vi "ES Main.vi"(10 "Data Type DVRs":T1, 11 "Config Folder":path) -> ()   [LabVIEW 2018]
uses:
  <vilib>/ORNL/CSEISMIC DDS/CSEISMIC DDS Base/Data Types/Controls/DeviceID.ctl
  Controls/DDS State.ctl
  Controls/Data Type DVRs.ctl
  Controls/Generation Mode Loop Selector.ctl
  <vilib>/ORNL/CSEISMIC DDS/CSEISMIC DDS Base/Data Types/DER_setGenerationMode.ctl
  <vilib>/ORNL/CSEISMIC DDS/CSEISMIC DDS Base/Data Types/Controls/Generation Mode.ctl
  Controls/GenerationMode.ctl
  <vilib>/ORNL/CSEISMIC DDS/CSEISMIC DDS Base/Data Types/IED_Status.ctl
  <vilib>/ORNL/CSEISMIC DDS/CSEISMIC DDS Base/Data Types/Controls/Timestamp.ctl
  <vilib>/ORNL/CSEISMIC DDS/CSEISMIC DDS Base/Data Types/DER_Control.ctl
  <vilib>/ORNL/CSEISMIC DDS/CSEISMIC DDS Base/Data Types/DER_SetPointP.ctl
  <vilib>/ORNL/CSEISMIC DDS/CSEISMIC DDS Base/Data Types/DER_SetPointQ.ctl
  <vilib>/ORNL/CSEISMIC DDS/CSEISMIC DDS Base/Data Types/DER_SetPointV.ctl
  <vilib>/ORNL/CSEISMIC DDS/CSEISMIC DDS Base/Data Types/DER_VF.ctl
  <vilib>/ORNL/CSEISMIC DDS/CSEISMIC DDS Base/Data Types/DER_SetPointF.ctl
  <vilib>/ORNL/CSEISMIC DDS/CSEISMIC DDS Base/Data Types/DER_Measurement.ctl
  <vilib>/ORNL/CSEISMIC DDS/CSEISMIC DDS Base/Data Types/DER_Status.ctl
  <vilib>/ORNL/CSEISMIC DDS/CSEISMIC DDS Base/Data Types/Controls/DroopCurve.ctl
  <vilib>/ORNL/CSEISMIC DDS/CSEISMIC DDS Base/Data Types/ES_Measurement.ctl
  c0909f76-96e0-496f-a6f7-ac9c3abfbcaa.vi
  7c59bdfa-a6d0-42ea-a36a-6a540bb37f3e.vi
  e95f3c18-e29d-40e4-94d7-6429cff7ece6.vi
  5e6c5b3f-77aa-4a8f-ba55-705d5b229056.vi
  7d30dc78-1fe7-43d0-be68-14ef1da03709.vi
  d3906dff-0d56-43f1-806b-b312a818046b.vi
  60710d3d-d05d-4e06-abc4-5833922697d4.vi
  d723711c-90b5-43fd-9837-430fe65d8763.vi
  2b29db2b-b629-43ef-99c9-7f779e92d8e6.vi
  fb202ae5-af77-46d5-8a34-636558cc811c.vi
  de1367b4-29ab-415d-92d0-7fa0fc6667ea.vi
  a8c78b73-a0ab-4721-a181-3ce0dcbdf431.vi
  9b782105-9e9e-450c-bef0-451d1281a5e4.vi
  04e9c7aa-85a8-4273-86f5-9355a9113040.vi
  f60448c4-0b4d-4df0-bc80-4b02817c393f.vi
  ae97810f-c92e-4387-8c39-39f975af07db.vi
  Global Variables/Stop (Global).vi
  Global Variables/Measurements (Global).vi
  Global Variables/DDS States (Global).vi
  Global Variables/Manual Control (Global).vi
  <vilib>/ORNL/CSEISMIC DDS/CSEISMIC DDS Base/CSEISMIC DDS.lvclass
panel:
  out "P_ref":sgl
  out "Q_ref":sgl
  out "P_meas":sgl
  out "Vf Control":bool
  out "Q_meas":sgl
  out "f_islanded":fxp<+,20,6>
  out "Vq_ref":sgl
  out "5038 Count":u32
  out "Is VF Device?":bool
  in  "Ramp Rate (W)":sgl=5000.0
  out "MicrogridID":u8
  out "Error in DDS Loop":bool
  out "DDS Loop error out":errorcluster
  out "DDS State":T2=enum."Shutdown"
  out "DDS loop time":u32=103
  out "DDS Indicators":T3
  out "Error in Generation Mode Loop":bool
  out "error out GenMode Loop":errorcluster
  out "DDS state m/c loop time":u32=100
  out "DeviceID":T4
  out "Enable INV A":bool
  out "SOC":dbl
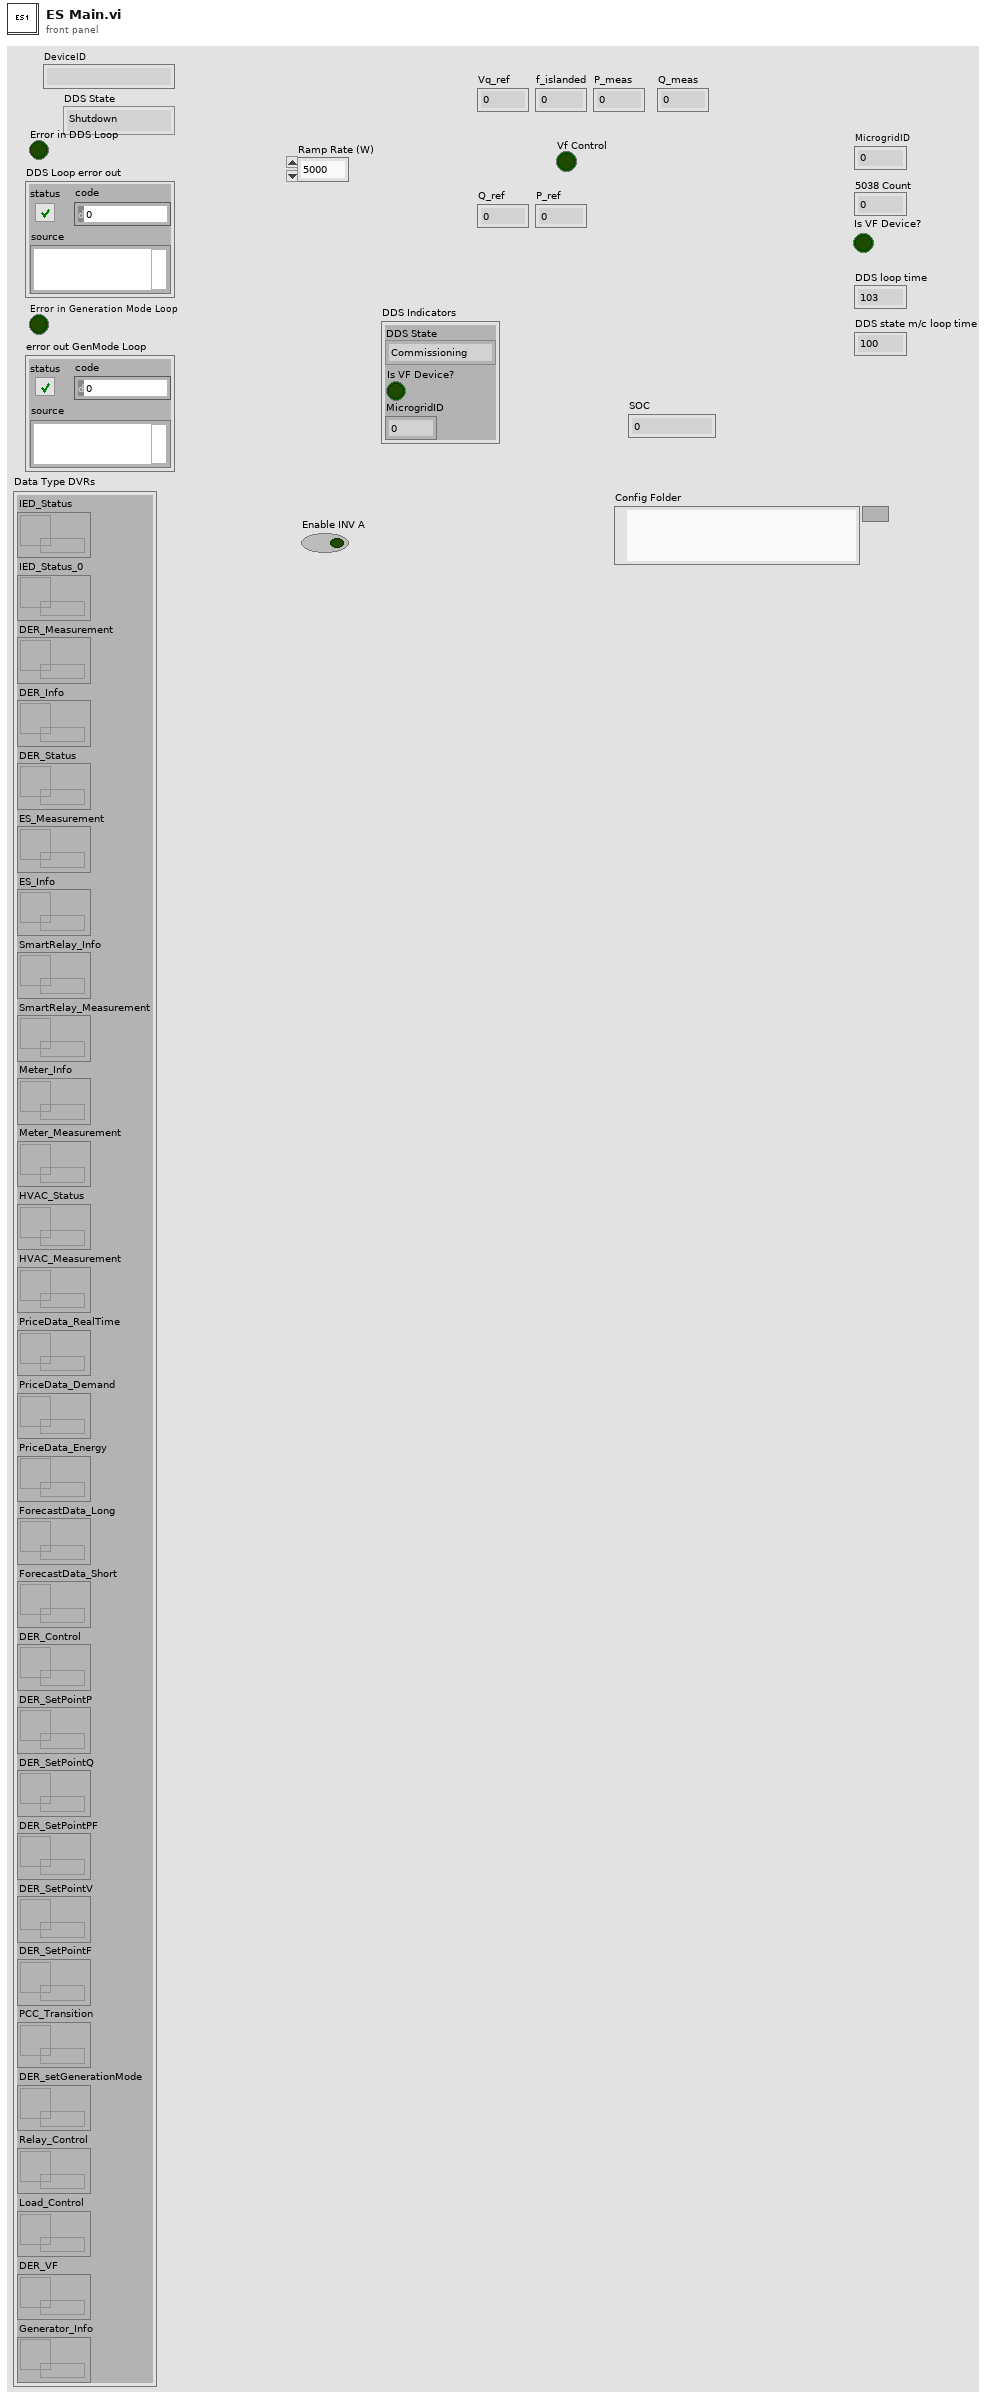
[diagram p1: front panel]
types:
  T1 = typedef "Data Type DVRs.ctl" = cluster{"IED_Status":refnum<data-value>, "IED_Status_0":refnum<data-value>, "DER_Measurement":refnum<data-value>, "DER_Info":refnum<data-value>, "DER_Status":refnum<data-value>, "ES_Measurement":refnum<data-value>, "ES_Info":refnum<data-value>, "SmartRelay_Info":refnum<data-value>, "SmartRelay_Measurement":refnum<data-value>, "Meter_Info":refnum<data-value>, "Meter_Measurement":refnum<data-value>, "HVAC_Status":refnum<data-value>, "HVAC_Measurement":refnum<data-value>, "PriceData_RealTime":refnum<data-value>, "PriceData_Demand":refnum<data-value>, "PriceData_Energy":refnum<data-value>, "ForecastData_Long":refnum<data-value>, "ForecastData_Short":refnum<data-value>, "DER_Control":refnum<data-value>, "DER_SetPointP":refnum<data-value>, "DER_SetPointQ":refnum<data-value>, "DER_SetPointPF":refnum<data-value>, "DER_SetPointV":refnum<data-value>, "DER_SetPointF":refnum<data-value>, "PCC_Transition":refnum<data-value>, "DER_setGenerationMode":refnum<data-value>, "Relay_Control":refnum<data-value>, "Load_Control":refnum<data-value>, "DER_VF":refnum<data-value>, "Generator_Info":refnum<data-value>}
  T2 = typedef "DDS State.ctl" = enum16{"Commissioning", "CheckID", "InitDDS", "ReadDDS", "WriteDDS", "CheckClose", "Close", "Shutdown"}
  T3 = cluster{"DDS State":T2, "Is VF Device?":bool, "MicrogridID":u8}
  T4 = typedef "CSEISMIC DDS.lvlib/CSEISMIC DDS.lvclass/DeviceID.ctl" = string
  T5 = typedef "Generation Mode Loop Selector.ctl" = enum16{"Commissioning", "Start", "Active", "VF Device", "Hold", "Close References", "Shutdown"}
  T6 = typedef "Scaling Coefficients Cluster.ctl" = cluster{"Measurements":T7, "Setpoints":T8}
  T7 = typedef "Scaling Coefficients Measurements.ctl" = cluster{"Current":dbl, "Voltage":dbl, "Real Power":dbl, "Reactive Power":dbl, "SOC":dbl}
  T8 = typedef "Scaling Coefficients Setpoints.ctl" = cluster{"Voltage":dbl, "Frequency":dbl, "Real Power":dbl, "Reactive Power":dbl}
  T9 = typedef "CSEISMIC DDS.lvlib/CSEISMIC DDS.lvclass/DER_Info.ctl" = cluster{"DeviceID":T4, "LineConfig":u8[], "NominalVoltage(V)":dbl, "PowerRating(kVA)":dbl, "VFControl":bool, "PControl":bool, "QControl":bool, "PFControl":bool, "PVControl":bool, "Droop":bool, "DroopConfigurable":bool, "Unbalanced":bool}
  T10 = typedef "CSEISMIC DDS.lvlib/CSEISMIC DDS.lvclass/ES_Info.ctl" = cluster{"DeviceID":T4, "EnergyRating (kWh)":dbl, "RampRate (kW/s)":dbl, "MaxPowerFactorLeading":dbl, "MaxPowerFactorLagging":dbl, "ChargingEfficiencyCurve":T11, "DischargingEfficiencyCurve":T11, "MinSOC (%)":dbl, "MaxSOC (%)":dbl}
  T11 = typedef "CSEISMIC DDS.lvlib/CSEISMIC DDS.lvclass/EfficiencyCurve.ctl" = cluster{"Power (kW)":dbl[], "Efficiency (%)":dbl[]}
  T12 = typedef "CSEISMIC DDS.lvlib/CSEISMIC DDS.lvclass/DER_setGenerationMode.ctl" = cluster{"DeviceID":T4, "Mode":T13}
  T13 = typedef "CSEISMIC DDS.lvlib/CSEISMIC DDS.lvclass/Generation Mode.ctl" = enum32{"Invalid", "PQ", "Droop", "PV", "PF", "VF"}
  T14 = typedef "GenerationMode.ctl" = enum32{"Invalid", "PQ", "Droop", "PV", "PF", "VF"}
  T15 = typedef "CSEISMIC DDS.lvlib/CSEISMIC DDS.lvclass/Timestamp.ctl" = cluster{"Seconds":u64, "Remainder":u64}
  T16 = typedef "CSEISMIC DDS.lvlib/CSEISMIC DDS.lvclass/IED_Status.ctl" = cluster{"DeviceID":T4, "Timestamp":T15, "MicrogridID":u8, "Active":bool, "Inactive":bool, "Error":i32, "Fault":bool, "ErrorString":string}
  T17 = typedef "CSEISMIC DDS.lvlib/CSEISMIC DDS.lvclass/DER_SetPointF.ctl" = cluster{"DeviceID":T4, "Frequency (Hz)":dbl}
  T18 = typedef "CSEISMIC DDS.lvlib/CSEISMIC DDS.lvclass/DER_VF.ctl" = cluster{"DeviceID":T4}
  T19 = typedef "CSEISMIC DDS.lvlib/CSEISMIC DDS.lvclass/DER_SetPointV.ctl" = cluster{"DeviceID":T4, "Voltage (V)":dbl}
  T20 = typedef "CSEISMIC DDS.lvlib/CSEISMIC DDS.lvclass/DER_SetPointQ.ctl" = cluster{"DeviceID":T4, "ReactivePower (kVAR)":dbl[]}
  T21 = typedef "CSEISMIC DDS.lvlib/CSEISMIC DDS.lvclass/DER_SetPointP.ctl" = cluster{"DeviceID":T4, "RealPower (kW)":dbl[]}
  T22 = typedef "CSEISMIC DDS.lvlib/CSEISMIC DDS.lvclass/DER_Control.ctl" = cluster{"DeviceID":T4, "Activate":bool, "Deactivate":bool}
  T23 = typedef "CSEISMIC DDS.lvlib/CSEISMIC DDS.lvclass/ES_Measurement.ctl" = cluster{"DeviceID":T4, "SOC (%)":dbl}
  T24 = typedef "CSEISMIC DDS.lvlib/CSEISMIC DDS.lvclass/DER_Status.ctl" = cluster{"DeviceID":T4, "VFControl":bool, "PControl":bool, "QControl":bool, "PFControl":bool, "PVControl":bool, "Droop":bool, "Unbalanced":bool, "MicrogridVF":bool, "RealDroop(kW)":T25, "ReactiveDroop(kVar)":T25}
  T25 = typedef "CSEISMIC DDS.lvlib/CSEISMIC DDS.lvclass/DroopCurve.ctl" = cluster{"XMin":dbl, "XMax":dbl, "YMin":dbl, "YMax":dbl}
  T26 = typedef "CSEISMIC DDS.lvlib/CSEISMIC DDS.lvclass/DER_Measurement.ctl" = cluster{"DeviceID":T4, "Voltage":dbl[], "Current":dbl[], "RealPower":dbl[], "ReactivePower":dbl[], "LineConfig":u8[], "Frequency":dbl}
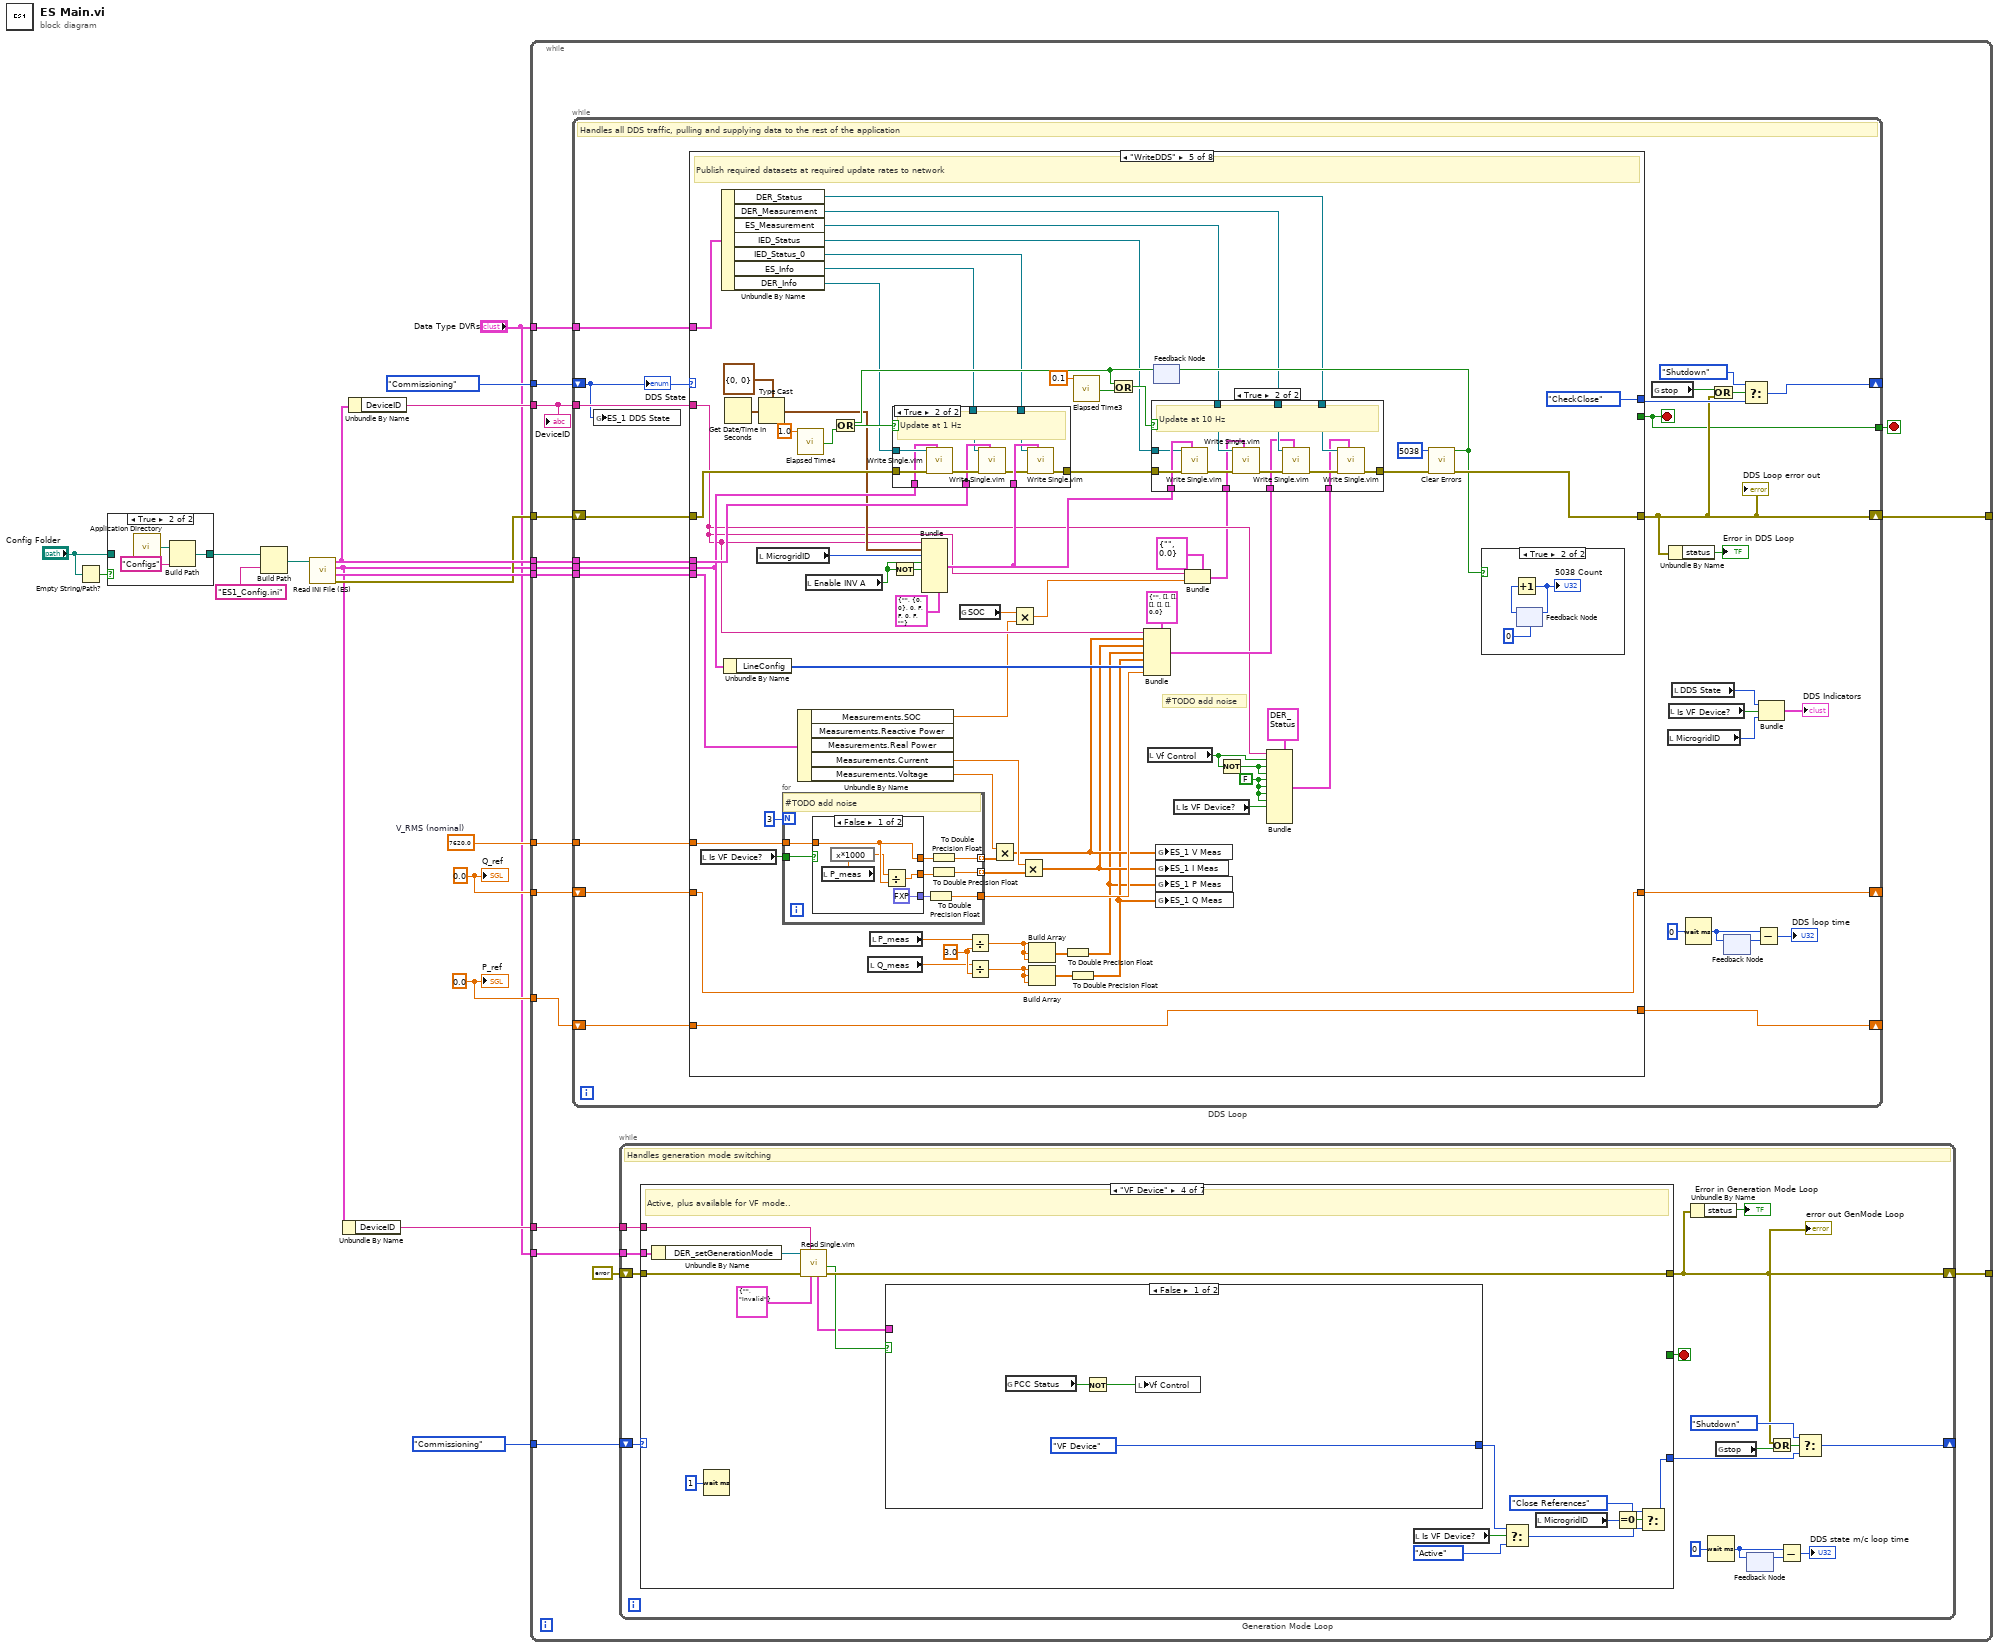
[diagram p0: block diagram]
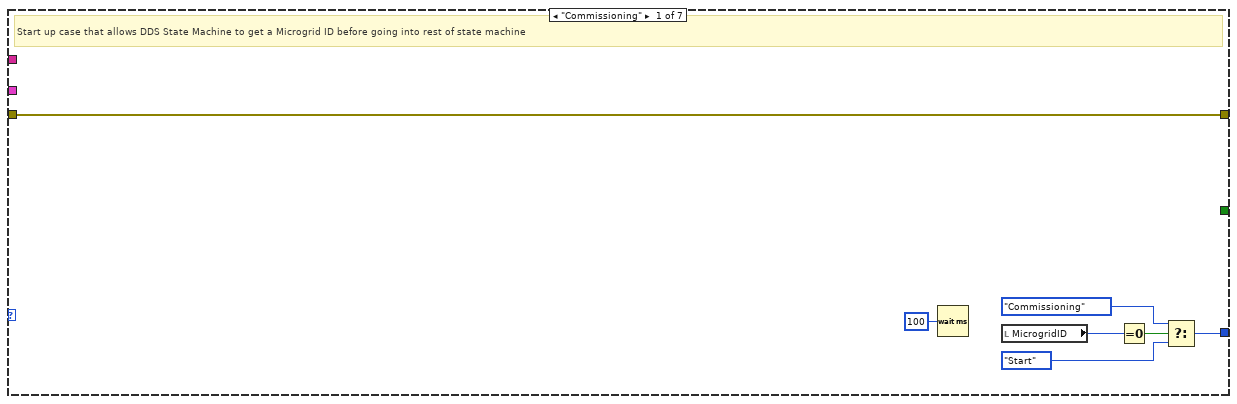
[diagram p2: hidden frame]
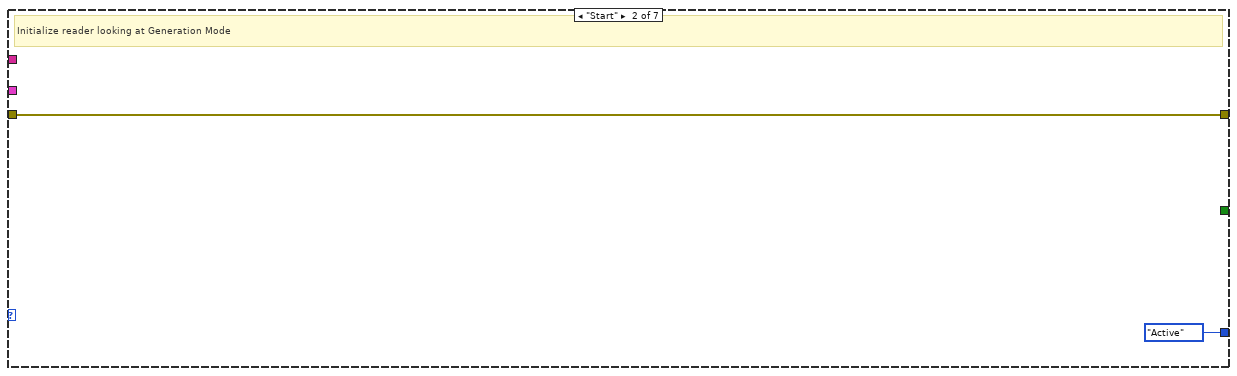
[diagram p3: hidden frame]
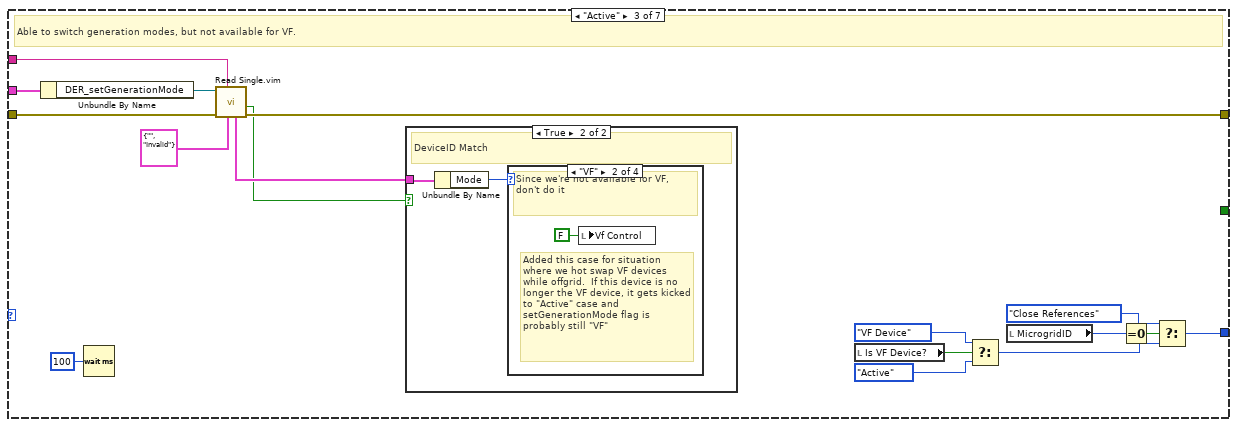
[diagram p4: hidden frame]
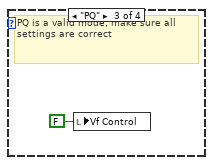
[diagram p7: hidden frame]
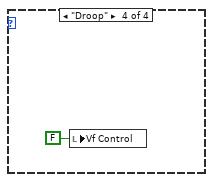
[diagram p8: hidden frame]
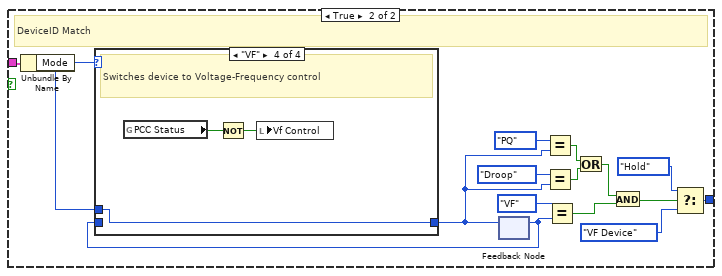
[diagram p9: hidden frame]
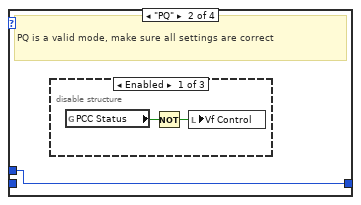
[diagram p11: hidden frame]
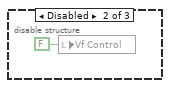
[diagram p12: hidden frame]
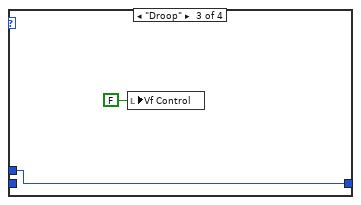
[diagram p14: hidden frame]
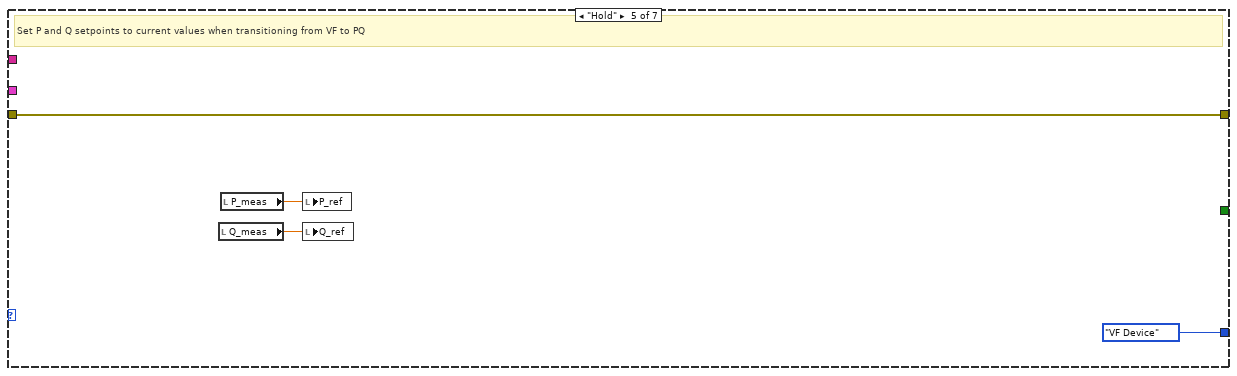
[diagram p15: hidden frame]
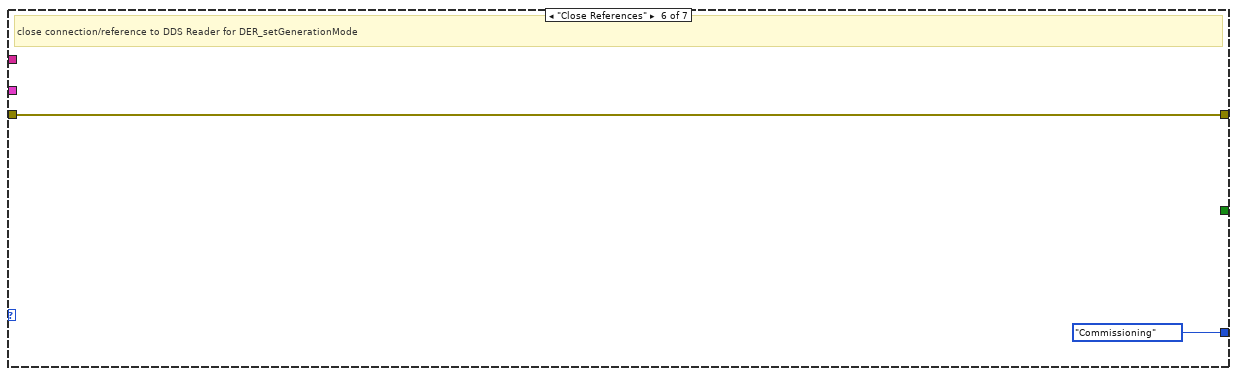
[diagram p16: hidden frame]
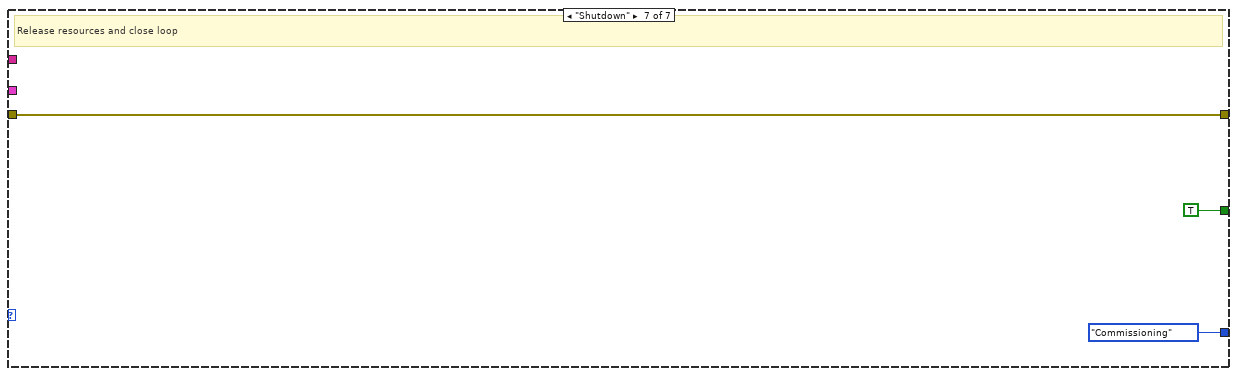
[diagram p17: hidden frame]
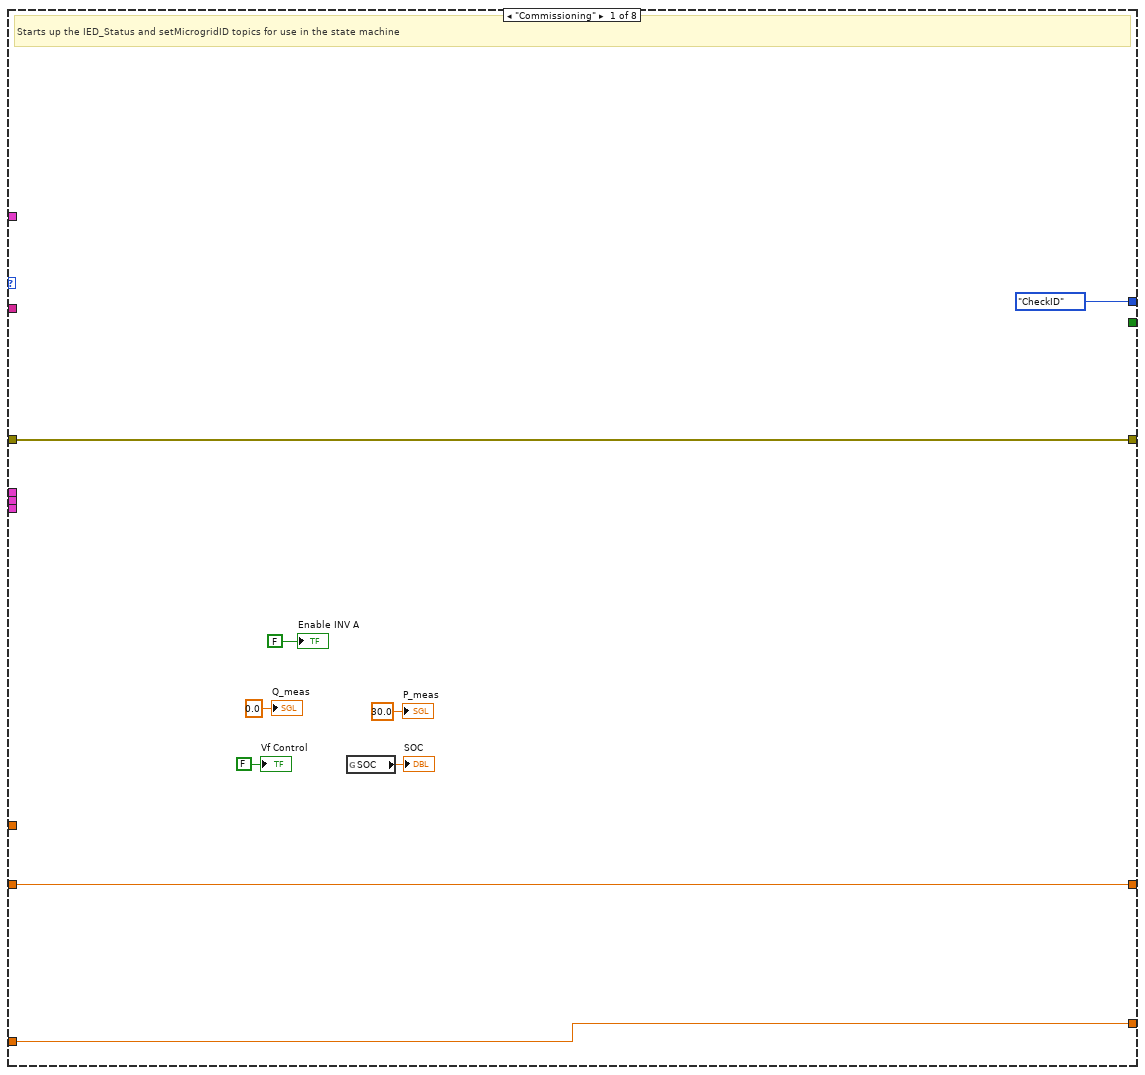
[diagram p18: hidden frame]
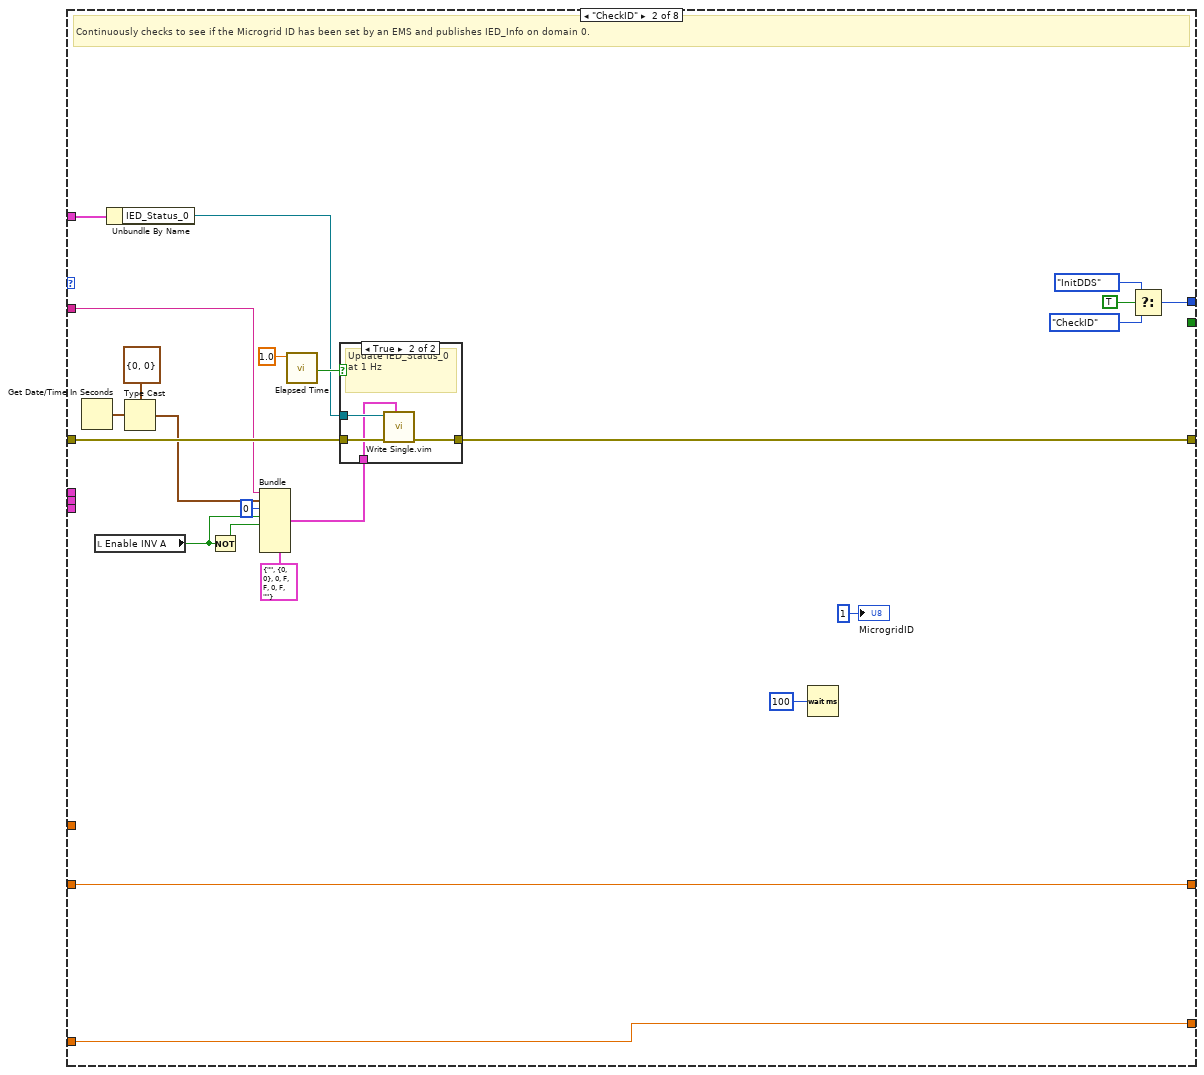
[diagram p19: hidden frame]
diagram:
  w5 = 7620.0  # V_RMS (nominal)
  w6 = sgl 0.0 ("Q_ref")
  w7 = sgl 0.0 ("P_ref")
  n1 = Empty String/Path?(string/path="Config Folder") -> (empty?=w4:bool)
  n2 = case shown="True" w4 {
    tunnel: [w18 w19] -> w2
    tunnel: "Config Folder" -> [w18 _]
    frame False {
    }
    frame True {
      n3 = call <vilib>:"Application Directory.vi"() -> ("Application Directory"=w21:path)
      n4 = Build Path(base path=w21, name or relative path="Configs") -> (appended path=w19:path)
    }
  }
  n5 = Build Path(base path=w2, name or relative path="ES1_Config.ini") -> (appended path=w16:path)
  n6 = call "Read INI File (ES).vi"("Path"=w16) -> ("error out"=w12:errorcluster, "Scaling Coefficients"=w13:T6, "DER_Info"=w10:T9, "ES_Info"=w14:T10)  [unwired: 7 in]
  n7 = Unbundle By Name(w10) -> ("DeviceID"=w11:T4)
  n8 = Unbundle By Name(w14) -> ("DeviceID"=w15:T4)
  n9 = while {
    tunnel: DDS_State."Commissioning" ("DDS State 2") -> [w38]
    tunnel: w10 -> [w37]
    tunnel: w12 -> [w36]
    tunnel: w13 -> [w35]
    tunnel: w15 -> [w34]
    tunnel: w14 -> [w33]
    tunnel: w11 -> [w31]
    tunnel: Generation_Mode_Loop_Selector."Commissioning" -> [w30]
    tunnel: [w29] -> _
    tunnel: [w28] -> _
    tunnel: w7 -> [w27]
    tunnel: w6 -> [w26]
    tunnel: w5 -> [w25]
    tunnel: "Data Type DVRs" -> [w24]
    tunnel: "Data Type DVRs" -> [w23]
    stop <- w32 stop-if-true
    n10 = while "DDS Loop" {
      shift-right: [w163] -> _
      shift-left: w38 -> [w140]
      tunnel: w34 -> [w167]
      shift-right: [w158] -> w28
      shift-left: w36 -> [w166]
      tunnel: w33 -> [w165]
      tunnel: w37 -> [w164]
      tunnel: w35 -> [w159]
      tunnel: [w156] -> w32
      shift-right: [w150] -> _
      shift-left: w27 -> [w149]
      shift-right: [w148] -> _
      shift-left: w26 -> [w147]
      tunnel: w25 -> [w142]
      tunnel: w24 -> [w151]
      stop <- w156 stop-if-true
      # "Handles all DDS traffic, pulling and supplying data to the rest of the application"
      n11 = global write "DDS States (Global).vi" "ES_1 DDS State"(w140) -> ()
      n12 = case shown="\"WriteDDS\"" w140 {
        tunnel: [DDS_State."CheckID" w194 DDS_State."ReadDDS" w254 DDS_State."CheckClose" w439 DDS_State."Commissioning" ("f") DDS_State."Commissioning" ("f")] -> w162
        tunnel: [w175 w185 w207 w221 w368 w438 w445 w452] -> w158
        tunnel: w167 -> [_ w184 _ w218 w353 _ _ _]
        tunnel: w166 -> [w175 w197 w207 w241 w387 w438 w445 w452]
        tunnel: w165 -> [_ _ _ _ w379 _ _ _]
        tunnel: w164 -> [_ _ _ _ w378 _ _ _]
        tunnel: [_ _ _ _ _ _ _ TRUE] -> w156
        tunnel: w159 -> [_ _ _ w210 w374 _ _ _]
        tunnel: w151 -> [_ w179 _ w242 w329 _ _ _]
        tunnel: [w174 w183 w206 w252 w346 w437 w443 w449] -> w150
        tunnel: w149 -> [w174 w183 w206 w251 w346 w437 w443 w449]
        tunnel: [w173 w182 w205 w249 w345 w436 w442 w448] -> w148
        tunnel: w147 -> [w173 w182 w205 w248 w345 w436 w442 w448]
        tunnel: w142 -> [_ _ _ _ w337 _ _ _]
        frame "Commissioning" {
          # "Starts up the IED_Status and setMicrogridID topics for use in the state machine"
          n13 = global read "Manual Control (Global).vi" "SOC"() -> (→"SOC":dbl)
          "Q_meas" <- sgl 0.0 ("Q_meas")
          "Vf Control" <- FALSE ("Vf Control")
          "P_meas" <- sgl 30.0 ("P_meas")
          "Enable INV A" <- FALSE ("Enable INV A")
        }
        frame "CheckID" {
          # "Continuously checks to see if the Microgrid ID has been set by an EMS and publishes IED_Info on domain 0."
          n14 = Get Date/Time In Seconds() -> (seconds since 1Jan1904=w190:timestamp)
          n15 = local read "Enable INV A"() -> (w181:bool)
          n16 = Unbundle By Name(w179) -> ("IED_Status_0"=w178:refnum<data-value>)
          n17 = Type Cast(type=T15 {"Seconds"=0, "Remainder"=0} ("Timestamp"), x=w190) -> (*(type *) &x=w188:T15)
          n18 = Not(x=w181) -> (.not. x?=w186:bool)
          n19 = Bundle(cluster=T16 {"DeviceID"="", "Timestamp"={"Seconds"=0, "Remainder"=0}, "MicrogridID"=0, "Active"=FALSE, "Inactive"=FALSE, "Error"=0, "Fault"=FALSE, "ErrorString"=""} ("output cluster"), "DeviceID"=w184, "Timestamp"=w188, "MicrogridID"=u8 0, "Active"=w181, "Inactive"=w186) -> (w198:T16)  [unwired: 3 in]
          n20 = call "Elapsed Time"("Time Target (s)"=1.0) -> ("Time has Elapsed"=w193:bool)  [unwired: 11 in, 7 out]
          n21 = case shown="True" w193 {
            tunnel: w198 -> [_ w201]
            tunnel: [w200 w202] -> w185
            tunnel: w197 -> [w200 w203]
            tunnel: w178 -> [_ w204]
            frame False {
            }
            frame True {
              # "Update IED_Status_0 at 1 Hz"
              n22 = call "Write Single.vim"("Data Element"=w201, "error in"=w203, "Data DVR"=w204) -> ("dup error out"=w202:errorcluster)  [unwired: 8 in]
            }
          }
          n23 = Wait (ms)(milliseconds to wait=u32 100) -> ()  [unwired: 1 out]
          n24 = Select(t=DDS_State."InitDDS", s=TRUE, f=DDS_State."CheckID") -> (s? t:f=w194:T2)
          "MicrogridID" <- u8 1 ("MicrogridID")
        }
        frame "InitDDS" {
          # "This initializes all readers and writers for DDS."
        }
        frame "ReadDDS" {
          # "Read device datasets from network and pass valid values to FPGA layer"
          n25 = Unbundle By Name(w242) -> ("DER_VF"=w217:refnum<data-value>, "DER_SetPointV"=w215:refnum<data-value>, "DER_SetPointF"=w226:refnum<data-value>, "DER_SetPointQ"=w230:refnum<data-value>, "DER_SetPointP"=w234:refnum<data-value>, "DER_Control"=w240:refnum<data-value>)
          n26 = call "Read Single.vim"("Data Type"=T22 {"DeviceID"="", "Activate"=FALSE, "Deactivate"=FALSE} ("DER_Control"), "DeviceID"=w218, "error in"=w241, "Data DVR"=w240) -> ("dup error out"=w236:errorcluster, "Valid"=w239:bool, "Data Element"=w238:T22)  [unwired: 5 in]
          n27 = call "Read Single.vim"("Data Type"=T21 {"DeviceID"="", "RealPower (kW)"=[]} ("DER_SetPointP"), "DeviceID"=w218, "error in"=w236, "Data DVR"=w234) -> ("dup error out"=w231:errorcluster, "Valid"=w233:bool, "Data Element"=w232:T21)  [unwired: 5 in]
          n28 = call "Read Single.vim"("Data Type"=T20 {"DeviceID"="", "ReactivePower (kVAR)"=[]} ("DER_SetPointQ"), "DeviceID"=w218, "error in"=w231, "Data DVR"=w230) -> ("dup error out"=w225:errorcluster, "Valid"=w228:bool, "Data Element"=w227:T20)  [unwired: 5 in]
          n29 = case shown="True" w233 {
            tunnel: w232 -> [_ w315]
            tunnel: w210 -> [_ w314]
            tunnel: [w295 w309] -> w252
            tunnel: w251 -> [w295 _]
            frame False {
              # "Non-matching DeviceID"
            }
            frame True {
              # "DeviceID matches this device"
              n30 = Unbundle By Name(w314) -> ("Setpoints.Real Power"=w312:dbl)
              n31 = Unbundle By Name(w315) -> ("RealPower (kW)"=w313:dbl[])
              n32 = global read "Measurements (Global).vi" "Load P Meas"() -> (w299:dbl[])
              n33 = global read "Measurements (Global).vi" "ES_2 P Meas"() -> (w303:dbl[])
              n34 = global read "Measurements (Global).vi" "Gen P Meas"() -> (w302:dbl[])
              n35 = global read "Measurements (Global).vi" "PV P Meas"() -> (w301:dbl[])
              n36 = Compound Arithmetic op=ADD(w303, w302, w301) -> (w300:dbl[])
              n37 = Add Array Elements(numeric array=w313) -> (sum=w311:dbl)
              n38 = Subtract(x=w300, y=w299) -> (x-y=w298:dbl[])
              n39 = Multiply(x=w312, y=w311) -> (x*y=w310:dbl)
              n40 = Add Array Elements(numeric array=w298) -> (sum=w296:dbl)
              n41 = local read "Enable INV A"() -> (w304:bool)
              n42 = local read "Vf Control"() -> (w305:bool)
              n43 = To Single Precision Float(number=w310) -> (single precision float=w307:sgl)
              n44 = To Single Precision Float(number=w296) -> (single precision float=w297:sgl)
              n45 = Select(t=w297, s=w305, f=w307) -> (s? t:f=w306:sgl)
              n46 = Select(t=w306, s=w304, f=sgl 0.0) -> (s? t:f=w309:sgl)
            }
          }
          n47 = case shown="True" w228 {
            tunnel: w227 -> [_ w294]
            tunnel: w210 -> [_ w293]
            tunnel: [w275 w285] -> w249
            tunnel: w248 -> [w275 _]
            frame False {
              # "Non-matching DeviceID"
            }
            frame True {
              # "DeviceID matches this device"
              n48 = Unbundle By Name(w293) -> ("Setpoints.Reactive Power"=w290:dbl)
              n49 = Unbundle By Name(w294) -> ("ReactivePower (kVAR)"=w292:dbl[])
              n50 = global read "Measurements (Global).vi" "Load Q Meas"() -> (w281:dbl[])
              n51 = global read "Measurements (Global).vi" "ES_2 Q Meas"() -> (w277:dbl[])
              n52 = global read "Measurements (Global).vi" "Gen Q Meas"() -> (w278:dbl[])
              n53 = global read "Measurements (Global).vi" "PV Q Meas"() -> (w279:dbl[])
              n54 = Compound Arithmetic op=ADD(w277, w278, w279) -> (w280:dbl[])
              n55 = Add Array Elements(numeric array=w292) -> (sum=w291:dbl)
              n56 = Subtract(x=w280, y=w281) -> (x-y=w282:dbl[])
              n57 = Multiply(x=w290, y=w291) -> (x*y=w289:dbl)
              n58 = Add Array Elements(numeric array=w282) -> (sum=w276:dbl)
              n59 = To Single Precision Float(number=w289) -> (single precision float=w288:sgl)
              n60 = local read "Enable INV A"() -> (w284:bool)
              n61 = local read "Vf Control"() -> (w283:bool)
              n62 = Select(t=w276, s=w283, f=w288) -> (s? t:f=w287:dbl)
              n63 = Select(t=w287, s=w284, f=sgl 0.0) -> (s? t:f=w285:dbl)
            }
          }
          n64 = call "Read Single.vim"("Data Type"=T17 {"DeviceID"="", "Frequency (Hz)"=0.0} ("DER_SetPointVF"), "DeviceID"=w218, "error in"=w225, "Data DVR"=w226) -> ("dup error out"=w214:errorcluster, "Valid"=w224:bool, "Data Element"=w223:T17)  [unwired: 5 in]
          n65 = call "Read Single.vim"("Data Type"=T19 {"DeviceID"="", "Voltage (V)"=0.0} ("DER_SetPointVF"), "DeviceID"=w218, "error in"=w214, "Data DVR"=w215) -> ("dup error out"=w213:errorcluster, "Valid"=w211:bool, "Data Element"=w209:T19)  [unwired: 5 in]
          n66 = case shown="True" w211 {
            tunnel: w210 -> [_ w260]
            tunnel: w209 -> [_ w259]
            frame False {
            }
            frame True {
              n67 = Unbundle By Name(w260) -> ("Setpoints.Voltage"=w257:dbl)
              n68 = Unbundle By Name(w259) -> ("Voltage (V)"=w258:dbl)
              n69 = Multiply(x=w258, y=w257) -> (x*y=w262:dbl)
              n70 = To Single Precision Float(number=w262) -> (single precision float=→"Vq_ref":sgl)
            }
          }
          n71 = case shown="True" w224 {
            tunnel: w223 -> [_ w274]
            tunnel: w210 -> [_ w273]
            frame False {
              # "Non-matching DeviceID"
            }
            frame True {
              # "DeviceID matches this device"
              n72 = Unbundle By Name(w273) -> ("Setpoints.Frequency"=w272:dbl)
              n73 = Unbundle By Name(w274) -> ("Frequency (Hz)"=w268:dbl)
              n74 = Multiply(x=w272, y=w268) -> (x*y=w270:dbl)
              n75 = To Fixed-Point(fixed-point type=fxp<+,20,6> 0.0 ("f_islanded"), number=w270) -> (fixed-point=→"f_islanded":fxp<+,20,6>)
            }
          }
          n76 = case shown="True" w239 {
            tunnel: w238 -> [_ w319]
            frame False {
              # "Non-matching DeviceID"
            }
            frame True {
              # "DeviceID matches this device"
              n77 = Unbundle By Name(w319) -> ("Activate"=w317:bool, "Deactivate"=w318:bool)
              n78 = Compound Arithmetic op=AND(w317, invert w318) -> (w316:bool)
              n79 = local write "Enable INV A"(w316) -> ()
            }
          }
          n80 = call "Read Single.vim"("Data Type"=T18 {"DeviceID"=""} ("DER_VF"), "DeviceID"=w218, "error in"=w213, "Data DVR"=w217) -> ("dup error out"=w221:errorcluster, "Valid"=w220:bool, "Data Element"=w219:T18)  [unwired: 5 in]
          n81 = local read "P_ref"() -> (w246:sgl)
          n82 = local read "Q_ref"() -> (w247:sgl)
          n83 = case shown="True" w220 {
            tunnel: w219 -> [_ w267]
            tunnel: w218 -> [_ w265]
            frame False {
              # "Non-matching DeviceID"
              n84 = local write "Is VF Device?"(FALSE ("Is VF Device?")) -> ()
            }
            frame True {
              # "DeviceID matches this device"
              n85 = Unbundle(w267) -> ("DeviceID"=w266:T4)
              n86 = Equal?(x=w265, y=w266) -> (x = y?=→"Is VF Device?":bool)
            }
          }
          n87 = call "Ramp Rate Coercion.vi"("Requested Value"=w252, "Original Value"=w246, "Ramp Rate (W)"="Ramp Rate (W)") -> ("Coerced Value"=w245:sgl)  [unwired: 8 in]
          n88 = local write "P_meas"(w245) -> ()
          n89 = local write "P_ref"(w245) -> ()
          n90 = call "Ramp Rate Coercion.vi"("Requested Value"=w249, "Original Value"=w247, "Ramp Rate (W)"="Ramp Rate (W)") -> ("Coerced Value"=w244:sgl)  [unwired: 8 in]
          n91 = local write "Q_meas"(w244) -> ()
          n92 = local write "Q_ref"(w244) -> ()
          n93 = Wait (ms)(milliseconds to wait=u32 100) -> ()  [unwired: 1 out]
          n94 = Select(t=DDS_State."Close", s=FALSE, f=DDS_State."WriteDDS") -> (s? t:f=w254:T2)
        }
        frame "WriteDDS" {
          w349 = sgl 3.0 ("y")
          w340 = FALSE ("PFControl")
          # "#TODO add noise"
          # "Publish required datasets at required update rates to network"
          n95 = local read "Is VF Device?"() -> (w338:bool)
          n96 = Unbundle By Name(w329) -> ("DER_Status"=w322:refnum<data-value>, "DER_Measurement"=w323:refnum<data-value>, "ES_Measurement"=w324:refnum<data-value>, "IED_Status"=w325:refnum<data-value>, "IED_Status_0"=w326:refnum<data-value>, "ES_Info"=w327:refnum<data-value>, "DER_Info"=w328:refnum<data-value>)
          n97 = Unbundle By Name(w378) -> ("LineConfig"=w377:u8[])
          n98 = Get Date/Time In Seconds() -> (seconds since 1Jan1904=w362:timestamp)
          n99 = local read "MicrogridID"() -> (w358:u8)
          n100 = Type Cast(type=T15 {"Seconds"=0, "Remainder"=0} ("Timestamp"), x=w362) -> (*(type *) &x=w359:T15)
          n101 = for {
            N: 3 -> [_]
            tunnel: [w399] -> w373 mode=indexing
            tunnel: [w398] -> w372 mode=indexing
            tunnel: w338 -> [w395]
            tunnel: w337 -> [w394]
            tunnel: [w393] -> w336
            # "#TODO add noise"
            n102 = case shown="False" w395 {
              tunnel: [w403 w408] -> w397
              tunnel: [w404 w409] -> w396
              tunnel: w394 -> [w403 _]
              tunnel: [fxp<+,20,6> 60.0 ("f_islanded") w407] -> w392
              frame False {
                n103 = local read "P_meas"() -> (w401:sgl)
                n104 = expression code="x*1000"(w401) -> (w400:sgl)
                n105 = Divide(x=w400, y=w403) -> (x/y=w404:dbl)
              }
              frame True {
                n106 = local read "P_meas"() -> (w406:sgl)
                n107 = local read "Vq_ref"() -> (w408:sgl)
                n108 = local read "f_islanded"() -> (w407:fxp<+,20,6>)
                n109 = expression code="x*1000"(w406) -> (w405:sgl)
                n110 = Divide(x=w405, y=w408) -> (x/y=w409:sgl)
              }
            }
            n111 = To Double Precision Float(number=w392) -> (double precision float=w393:dbl)
            n112 = To Double Precision Float(number=w397) -> (double precision float=w399:dbl)
            n113 = To Double Precision Float(number=w396) -> (double precision float=w398:dbl)
          }
          n114 = call "Elapsed Time4"("Time Target (s)"=1.0) -> ("Time has Elapsed"=w375:bool)  [unwired: 11 in, 7 out]
          n115 = Unbundle By Name(w374) -> ("Measurements.SOC"=w350:dbl, "Measurements.Current"=w370:dbl, "Measurements.Voltage"=w371:dbl)  [unwired: 2 out]
          n116 = local read "Enable INV A"() -> (w344:bool)
          n117 = local read "Q_meas"() -> (w343:sgl)
          n118 = local read "P_meas"() -> (w321:sgl)
          n119 = Not(x=w344) -> (.not. x?=w357:bool)
          n120 = Bundle(cluster=T16 {"DeviceID"="", "Timestamp"={"Seconds"=0, "Remainder"=0}, "MicrogridID"=0, "Active"=FALSE, "Inactive"=FALSE, "Error"=0, "Fault"=FALSE, "ErrorString"=""} ("IED_Status"), "DeviceID"=w353, "Timestamp"=w359, "MicrogridID"=w358, "Active"=w344, "Inactive"=w357) -> (w385:T16)  [unwired: 3 in]
          n121 = global read "Manual Control (Global).vi" "SOC"() -> (w320:dbl)
          n122 = Divide(x=w321, y=w349) -> (x/y=w348:sgl)
          n123 = Divide(x=w343, y=w349) -> (x/y=w347:sgl)
          n124 = Multiply(x=w371, y=w373) -> (x*y=w335:dbl[])
          n125 = Multiply(x=w320, y=w350) -> (x*y=w351:dbl)
          n126 = Multiply(x=w370, y=w372) -> (x*y=w334:dbl[])
          n127 = Build Array(w348, w348, w348) -> (w333:sgl[])
          n128 = Build Array(w347, w347, w347) -> (w332:sgl[])
          n129 = To Double Precision Float(number=w333) -> (double precision float=w330:dbl[])
          n130 = To Double Precision Float(number=w332) -> (double precision float=w331:dbl[])
          n131 = call "Elapsed Time3"("Time Target (s)"=0.1) -> ("Time has Elapsed"=w380:bool)  [unwired: 11 in, 7 out]
          n132 = Bundle(cluster=T26 {"DeviceID"="", "Voltage"=[], "Current"=[], "RealPower"=[], "ReactivePower"=[], "LineConfig"=[], "Frequency"=0.0} ("DER_Measurement"), "DeviceID"=w353, "Voltage"=w335, "Current"=w334, "RealPower"=w330, "ReactivePower"=w331, "LineConfig"=w377, "Frequency"=w336) -> (w384:T26)
          n133 = local read "Vf Control"() -> (w342:bool)
          n134 = feedback #1() -> (w364:bool)  [unwired: 1 in]
          n135 = Or(x=w364, y=w375) -> (x .or. y?=w366:bool)
          n136 = case shown="True" w366 {
            tunnel: w387 -> [w424 w434]
            tunnel: [w424 w427] -> w386
            tunnel: w385 -> [_ w429]
            tunnel: w379 -> [_ w430]
            tunnel: w378 -> [_ w432]
            tunnel: w328 -> [_ w433]
            tunnel: w327 -> [_ w426]
            tunnel: w326 -> [_ w425]
            frame False {
            }
            frame True {
              # "Update at 1 Hz"
              n137 = call "Write Single.vim"("Data Element"=w432, "error in"=w434, "Data DVR"=w433) -> ("dup error out"=w431:errorcluster)  [unwired: 8 in]
              n138 = call "Write Single.vim"("Data Element"=w430, "error in"=w431, "Data DVR"=w426) -> ("dup error out"=w428:errorcluster)  [unwired: 8 in]
              n139 = call "Write Single.vim"("Data Element"=w429, "error in"=w428, "Data DVR"=w425) -> ("dup error out"=w427:errorcluster)  [unwired: 8 in]
            }
          }
          n140 = Or(x=w364, y=w380) -> (x .or. y?=w365:bool)
          n141 = global write "Measurements (Global).vi" "ES_1 V Meas"(w335) -> ()
          n142 = global write "Measurements (Global).vi" "ES_1 I Meas"(w334) -> ()
          n143 = global write "Measurements (Global).vi" "ES_1 P Meas"(w330) -> ()
          n144 = global write "Measurements (Global).vi" "ES_1 Q Meas"(w331) -> ()
          n145 = local read "Is VF Device?"() -> (w369:bool)
          n146 = Bundle(cluster=T23 {"DeviceID"="", "SOC (%)"=0.0} ("ES_Measurement"), "DeviceID"=w353, "SOC (%)"=w351) -> (w352:T23)
          n147 = Not(x=w342) -> (.not. x?=w341:bool)
          n148 = Bundle(cluster=T24 {"DeviceID"="", "VFControl"=FALSE, "PControl"=FALSE, "QControl"=FALSE, "PFControl"=FALSE, "PVControl"=FALSE, "Droop"=FALSE, "Unbalanced"=FALSE, "MicrogridVF"=FALSE, "RealDroop(kW)"={"XMin"=0.0, "XMax"=0.0, "YMin"=0.0, "YMax"=0.0}, "ReactiveDroop(kVar)"={"XMin"=0.0, "XMax"=0.0, "YMin"=0.0, "YMax"=0.0}} ("DER_Status"), "DeviceID"=w353, "VFControl"=w342, "PControl"=w341, "QControl"=w341, "PFControl"=w340, "PVControl"=w340, "Droop"=w340, "Unbalanced"=w340, "MicrogridVF"=w369) -> (w383:T24)  [unwired: 2 in]
          n149 = case shown="True" w365 {
            tunnel: w325 -> [_ w421]
            tunnel: w386 -> [w410 w423]
            tunnel: w385 -> [_ w422]
            tunnel: w384 -> [_ w415]
            tunnel: w383 -> [_ w412]
            tunnel: [w410 w411] -> w382
            tunnel: w352 -> [_ w418]
            tunnel: w324 -> [_ w419]
            tunnel: w323 -> [_ w416]
            tunnel: w322 -> [_ w413]
            frame False {
            }
            frame True {
              # "Update at 10 Hz"
              n150 = call "Write Single.vim"("Data Element"=w422, "error in"=w423, "Data DVR"=w421) -> ("dup error out"=w420:errorcluster)  [unwired: 8 in]
              n151 = call "Write Single.vim"("Data Element"=w418, "error in"=w420, "Data DVR"=w419) -> ("dup error out"=w417:errorcluster)  [unwired: 8 in]
              n152 = call "Write Single.vim"("Data Element"=w415, "error in"=w417, "Data DVR"=w416) -> ("dup error out"=w414:errorcluster)  [unwired: 8 in]
              n153 = call "Write Single.vim"("Data Element"=w412, "error in"=w414, "Data DVR"=w413) -> ("dup error out"=w411:errorcluster)  [unwired: 8 in]
            }
          }
          n154 = call <vilib>:"Clear Errors.vi"("error in (no error)"=w382, "specific error code to clear (0: all)"=5038) -> ("error out"=w368:errorcluster, "specific error cleared?"=w363:bool)  [unwired: 4 in]
          n155 = feedback-in #1(w363) -> ()
          n156 = case shown="True" w363 {
            frame False {
            }
            frame True {
              n157 = feedback #2(u32 0 ("5038 Count")) -> (w390:u32)
              n158 = Increment(x=w390) -> (x+1=w391:u32)
              "5038 Count" <- w391
              n159 = feedback-in #2(w391) -> ()
            }
          }
        }
        frame "CheckClose" {
          # "Check to see if MicrogridID has been reset to 0, releasing the device from Microgrid control"
          n160 = Select(t=DDS_State."Close", s=FALSE, f=DDS_State."ReadDDS") -> (s? t:f=w439:T2)
        }
        frame "Close" {
          # "Set MicrogridID to 0 in order for Generation Mode Loop to function correctly."
          # "Deactivate the device"
          # "Release resources associated with microgrid ID, deactivate device, and return to CheckID state"
          n161 = flat-sequence {
            frame #0 {
              # "disables output"
              n162 = local write "Enable INV A"(FALSE ("PWM Enabled")) -> ()
            }
          }
          n163 = local write "MicrogridID"(u8 0 ("MicrogridID")) -> ()
        }
        frame "Shutdown" {
          # "Set MicrogridID to 0 in order for Generation Mode Loop to function correctly."
          # "Deactivate the device"
          # "Release resources and stop loop"
          n164 = flat-sequence {
            frame #0 {
              # "disables output"
              n165 = local write "Enable INV A"(FALSE ("PWM Enabled")) -> ()
            }
          }
          n166 = local write "MicrogridID"(u8 0 ("MicrogridID")) -> ()
        }
      }
      "DDS Loop error out" <- w158
      n167 = global read "Stop (Global).vi" "stop"() -> (w141:bool)
      n168 = local read "MicrogridID"() -> (w145:u8)
      n169 = local read "Is VF Device?"() -> (w144:bool)
      n170 = Unbundle By Name(w158) -> ("status"=→"Error in DDS Loop":bool)
      n171 = local read "DDS State"() -> (w143:T2)
      n172 = Wait (ms)(milliseconds to wait=u32 0) -> (millisecond timer value=w154:u32)
      n173 = Or(x=w141, y=w158) -> (x .or. y?=w160:bool)
      n174 = feedback #3() -> (w153:u32)  [unwired: 1 in]
      n175 = feedback-in #3(w154) -> ()
      n176 = Select(t=DDS_State."Shutdown", s=w160, f=w162) -> (s? t:f=w163:T2)
      n177 = Subtract(x=w154, y=w153) -> (x-y=→"DDS loop time":u32)
      n178 = Bundle("DDS State"=w143, "Is VF Device?"=w144, "MicrogridID"=w145) -> (→"DDS Indicators":T3)  [unwired: 1 in]
      "DDS State" <- w140
    }
    n179 = while "Generation Mode Loop" {
      shift-right: [w51] -> _
      shift-left: w30 -> [w54]
      shift-right: [w45] -> w29
      shift-left: errorcluster {"status"=FALSE, "code"=0, "source"=""} ("error out") -> [w49]
      tunnel: w31 -> [w47]
      tunnel: w23 -> [w50]
      stop <- w44 stop-if-true
      # "Handles generation mode switching"
      n180 = case shown="\"VF Device\"" w54 {
        tunnel: [w56 Generation_Mode_Loop_Selector."Active" w73 w96 Generation_Mode_Loop_Selector."VF Device" Generation_Mode_Loop_Selector."Commissioning" Generation_Mode_Loop_Selector."Commissioning"] -> w52
        tunnel: [_ _ _ _ _ _ TRUE] -> w44
        tunnel: w50 -> [_ _ w69 w93 _ _ _]
        tunnel: w49 -> [w55 w62 w67 w92 w133 w135 w138]
        tunnel: [w55 w62 w66 w91 w133 w135 w138] -> w45
        tunnel: w47 -> [_ _ w68 w86 _ _ _]
        frame "Commissioning" {
          # "Start up case that allows DDS State Machine to get a Microgrid ID before going into rest of state machine"
          n181 = Wait (ms)(milliseconds to wait=u32 100) -> ()  [unwired: 1 out]
          n182 = local read "MicrogridID"() -> (w60:u8)
          n183 = Equal To 0?(x=w60) -> (x = 0?=w59:bool)
          n184 = Select(t=Generation_Mode_Loop_Selector."Commissioning", s=w59, f=Generation_Mode_Loop_Selector."Start") -> (s? t:f=w56:T5)
        }
        frame "Start" {
          # "Initialize reader looking at Generation Mode"
        }
        frame "Active" {
          # "Able to switch generation modes, but not available for VF."
          n185 = Unbundle By Name(w69) -> ("DER_setGenerationMode"=w71:refnum<data-value>)
          n186 = Wait (ms)(milliseconds to wait=u32 100) -> ()  [unwired: 1 out]
          n187 = call "Read Single.vim"("Data Type"=T12 {"DeviceID"="", "Mode"=enum."Invalid"} ("DER_setGenerationMode"), "DeviceID"=w68, "error in"=w67, "Data DVR"=w71) -> ("dup error out"=w66:errorcluster, "Valid"=w64:bool, "Data Element"=w65:T12)  [unwired: 5 in]
          n188 = case shown="True" w64 {
            tunnel: w65 -> [_ w82]
            frame False {
            }
            frame True {
              # "DeviceID Match"
              n189 = Unbundle By Name(w82) -> ("Mode"=w81:T13)
              n190 = case shown="\"VF\"" w81 {
                frame "Invalid", Default {
                }
                frame "VF" {
                  # "Added this case for situation where we hot swap VF devices while offgrid.  If this device is no longer the VF device, it gets kicked to \"Active\" case and setGenerationMode flag is probably still \"VF\""
                  # "Since we're not available for VF, don't do it"
                  n191 = local write "Vf Control"(FALSE ("Vf Control")) -> ()
                }
                frame "PQ" {
                  # "PQ is a valid mode, make sure all settings are correct"
                  n192 = local write "Vf Control"(FALSE ("Vf Control")) -> ()
                }
                frame "Droop" {
                  n193 = local write "Vf Control"(FALSE ("Vf Control")) -> ()
                }
              }
            }
          }
          n194 = local read "Is VF Device?"() -> (w75:bool)
          n195 = Select(t=Generation_Mode_Loop_Selector."VF Device", s=w75, f=Generation_Mode_Loop_Selector."Active") -> (s? t:f=w74:T5)
          n196 = local read "MicrogridID"() -> (w80:u8)
          n197 = Equal To 0?(x=w80) -> (x = 0?=w79:bool)
          n198 = Select(t=Generation_Mode_Loop_Selector."Close References", s=w79, f=w74) -> (s? t:f=w73:T5)
        }
        frame "VF Device" {
          # "Active, plus available for VF mode.."
          n199 = Unbundle By Name(w93) -> ("DER_setGenerationMode"=w90:refnum<data-value>)
          n200 = Wait (ms)(milliseconds to wait=u32 1) -> ()  [unwired: 1 out]
          n201 = call "Read Single.vim"("Data Type"=T12 {"DeviceID"="", "Mode"=enum."Invalid"} ("DER_setGenerationMode"), "DeviceID"=w86, "error in"=w92, "Data DVR"=w90) -> ("dup error out"=w91:errorcluster, "Valid"=w88:bool, "Data Element"=w87:T12)  [unwired: 5 in]
          n202 = case shown="False" w88 {
            tunnel: w87 -> [_ w120]
            tunnel: [Generation_Mode_Loop_Selector."VF Device" w106] -> w94
            frame False {
              n203 = global read "Measurements (Global).vi" "PCC Status"() -> (w104:bool)
              n204 = Not(x=w104) -> (.not. x?=w103:bool)
              n205 = local write "Vf Control"(w103) -> ()
            }
            frame True {
              # "DeviceID Match"
              n206 = Unbundle By Name(w120) -> ("Mode"=w119:T13)
              n207 = feedback #4() -> (w113:T13)  [unwired: 1 in]
              n208 = case shown="\"VF\"" w119 {
                tunnel: w119 -> [_ w122 w127 w130]
                tunnel: [w121 w122 w127 w130] -> w118
                tunnel: w113 -> [w121 _ _ _]
                frame "Invalid", Default {
                }
                frame "PQ" {
                  # "PQ is a valid mode, make sure all settings are correct"
                  n209 = disable-structure shown="Enabled" {
                    frame Enabled {
                      n210 = global read "Measurements (Global).vi" "PCC Status"() -> (w124:bool)
                      n211 = Not(x=w124) -> (.not. x?=w123:bool)
                      n212 = local write "Vf Control"(w123) -> ()
                    }
                    frame Disabled {
                      n213 = local write "Vf Control"(FALSE ("Vf Control")) -> ()
                    }
                    frame Disabled {
                    }
                  }
                }
                frame "Droop" {
                  n214 = local write "Vf Control"(FALSE ("Vf Control")) -> ()
                }
                frame "VF" {
                  # "Switches device to Voltage-Frequency control"
                  n215 = global read "Measurements (Global).vi" "PCC Status"() -> (w129:bool)
                  n216 = Not(x=w129) -> (.not. x?=w128:bool)
                  n217 = local write "Vf Control"(w128) -> ()
                }
              }
              n218 = feedback-in #4(w118) -> ()
              n219 = Equal?(x=GenerationMode."PQ", y=w118) -> (x = y?=w115:bool)
              n220 = Equal?(x=GenerationMode."Droop", y=w118) -> (x = y?=w114:bool)
              n221 = Equal?(x=GenerationMode."VF", y=w113) -> (x = y?=w110:bool)
              n222 = Or(x=w115, y=w114) -> (x .or. y?=w111:bool)
              n223 = And(x=w111, y=w110) -> (x .and. y?=w109:bool)
              n224 = Select(t=Generation_Mode_Loop_Selector."Hold", s=w109, f=Generation_Mode_Loop_Selector."VF Device") -> (s? t:f=w106:T5)
            }
          }
          n225 = local read "Is VF Device?"() -> (w98:bool)
          n226 = Select(t=w94, s=w98, f=Generation_Mode_Loop_Selector."Active") -> (s? t:f=w97:T5)
          n227 = local read "MicrogridID"() -> (w102:u8)
          n228 = Equal To 0?(x=w102) -> (x = 0?=w101:bool)
          n229 = Select(t=Generation_Mode_Loop_Selector."Close References", s=w101, f=w97) -> (s? t:f=w96:T5)
        }
        frame "Hold" {
          # "Set P and Q setpoints to current values when transitioning from VF to PQ"
          n230 = local read "Q_meas"() -> (w131:sgl)
          n231 = local read "P_meas"() -> (w132:sgl)
          n232 = local write "P_ref"(w132) -> ()
          n233 = local write "Q_ref"(w131) -> ()
        }
        frame "Close References" {
          # "close connection/reference to DDS Reader for DER_setGenerationMode"
        }
        frame "Shutdown" {
          # "Release resources and close loop"
        }
      }
      "error out GenMode Loop" <- w45
      n234 = Unbundle By Name(w45) -> ("status"=→"Error in Generation Mode Loop":bool)
      n235 = Wait (ms)(milliseconds to wait=u32 0) -> (millisecond timer value=w42:u32)
      n236 = global read "Stop (Global).vi" "stop"() -> (w39:bool)
      n237 = feedback #5() -> (w41:u32)  [unwired: 1 in]
      n238 = feedback-in #5(w42) -> ()
      n239 = Or(x=w45, y=w39) -> (x .or. y?=w48:bool)
      n240 = Subtract(x=w42, y=w41) -> (x-y=→"DDS state m/c loop time":u32)
      n241 = Select(t=Generation_Mode_Loop_Selector."Shutdown", s=w48, f=w52) -> (s? t:f=w51:T5)
    }
    "DeviceID" <- w34
  }
  "Q_ref" <- w6
  "P_ref" <- w7
